vi "create_core.vi"() -> ()   [LabVIEW 2017, in "lvfase.lvclass"]
uses:
  lvfase.lvclass
panel:
  out "lvfase out":refnum<class "lvfase.lvclass">
  in  "lvfase in":refnum<class "lvfase.lvclass">
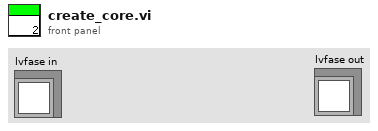
[diagram p1: front panel]
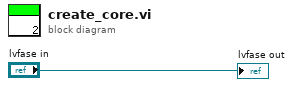
[diagram p0: block diagram]
diagram:
  "lvfase out" <- "lvfase in"
